vi "MyRIO Lidar Close.vi"(8 "error in (no error)":errorcluster) -> (0 "error out":errorcluster)   [LabVIEW 2016]
uses:
  Variables/MyRIO Lidar Class Data.vi
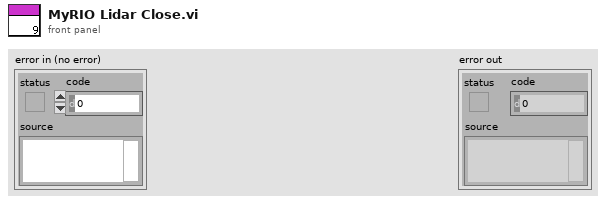
[diagram p1: front panel]
types:
  T1 = cluster{"Shared library path":path, "File Descriptor":i32}
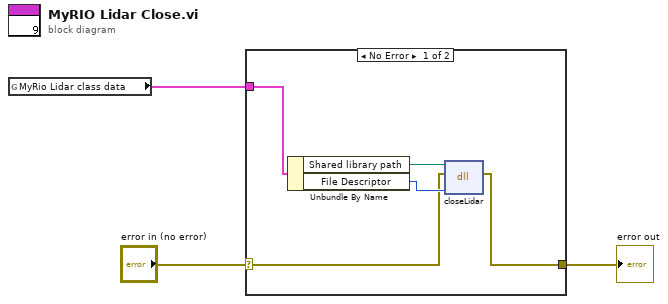
[diagram p0: block diagram]
diagram:
  n1 = global read "MyRIO Lidar Class Data.vi" "MyRio Lidar class data"() -> (w1:T1)
  n2 = case shown="No Error" "error in (no error)" {
    selector: "error in (no error)" -> [w5 w9]
    tunnel: [w4 w9] -> w2
    tunnel: w1 -> [w8 _]
    frame No Error {
      n3 = Unbundle By Name(w8) -> ("Shared library path"=w7:path, "File Descriptor"=w6:i32)
      n4 = dll-call lib="?" fn="closeLidar"(path in=w7, error in=w5, "fd"=w6) -> (error out=w4:errorcluster)  [unwired: 3 in, 1 out]
    }
    frame Error {
    }
  }
  "error out" <- w2
